vi "RT Main v1.0.vi"() -> ()   [LabVIEW 2017]
doc: "Changelog:\n\nv0.9:\n- Autocycle"
uses:
  Controls/Auto Delays.ctl
  support/Controls/All Inputs.ctl
  support/Controls/Index Details.ctl
  support/Controls/Auto Stats.ctl
  Controls/Auto Times.ctl
  Global Variables/RT GV.vi
  support/Message Queue/Enqueue Message (Single).vi
  Global Variables/FPGA GV.vi
  <vilib>/Utility/error.llb/Error Cluster From Error Code.vi
  <vilib>/rvi/errors/niLvFpgaAdjustHostInterfaceError.vi
  Global Variables/Network Globals.vi
  <vilib>/FPGAPlugInAG/Dynamic/niLvFpga_Close_Dynamic.vi
  <vilib>/rvi/interface/nirviReadWriteControl/nirviReadWriteControl.xnode
  Controls/FPGA Ref.ctl
  <vilib>/rvi/interface/nirviCloseFPGA/nirviCloseFPGA.xnode
  support/Message Queue/Message Queue.lvlib
  NiFpgaLv.dll
  <vilib>/rvi/interface/Simulation/niFpgaSimulationCallBeginRW.vi
panel:
  in  "Auto Para":T1={"Agitator Delays"=[250, 350], "TF Delays"=[700, 800, 2], "Insertion Delays"=[100, 500], "Cutting Delays"=[300, 300, 100], "PF Delays"=[250, 30000], "Measur. Delays"=[500.0, 188.9, 1.0], "Reject Delays"=[500], "BF Delays"=[1000, 1000]}
  in  "Stop Button 4":bool
  out "error out":errorcluster
  out "Wrong Message":string
  in  "Stop Button":bool
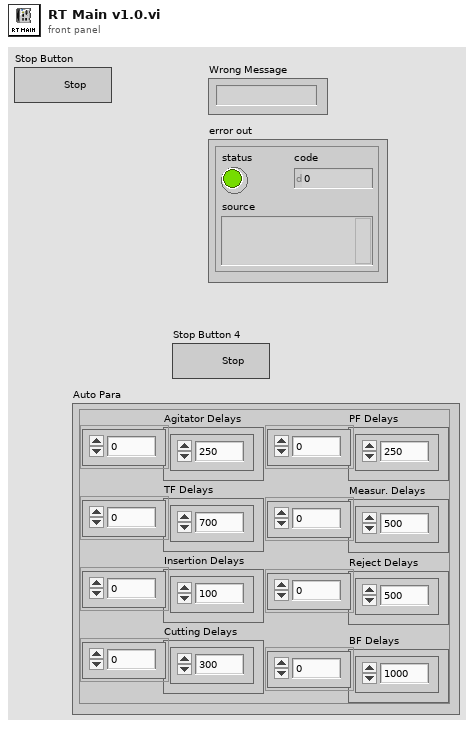
[diagram p1: front panel]
types:
  T1 = typedef "Auto Delays.ctl" = cluster{"Agitator Delays":u32[], "TF Delays":u32[], "Insertion Delays":u32[], "Cutting Delays":u32[], "PF Delays":u32[], "Measur. Delays":dbl[], "Reject Delays":u32[], "BF Delays":u32[]}
  T2 = typedef "FPGA Ref.ctl" = refnum<k20>
  T3 = cluster{"TL_Red":bool, "TL_Orange":bool, "TL_Green":bool, "TL_Buzzer":bool, "SOL_Index_Rotary_CW":bool, "SOL_Index_CNVR_Rotary_CCW":bool, "SOL_Index_CNVR_Stopper_Rear":bool, "SOL_Index_CNVR_Output _Separator _Rear":bool, "Bowl  Feeder_ ON":bool, "Pump_CNVR_Motor _ON":bool, "SOL_Gating_CYL_Rear":bool, "SOL_Tube_Feed_Agitatator":bool, "SOL_Tube_Feed_Gating_CYL":bool, "SOL_Insertion _CYL":bool, "SOL_Insertion_Clamp_CYL":bool, "SOL_Cutting_CYL":bool, "SOL_Cutting_Clamp_CYL":bool, "SOL_Insertion_Air_Nozzle":bool, "SOL_Measurement_CYL":bool, "SOL_Measure_Clamp_CYL":bool, "SOL_Rejection CYL_1":bool, "SOL_Rejection CYL_2":bool, "SOL_Rejection CYL_3":bool, "SOL_Rejection CYL_4":bool, "DO1.24":bool, "DO1.25":bool, "DO1.26":bool, "DO1.27":bool, "DO1.28":bool, "DO1.29":bool, "DO1.30":bool, "DO1.31":bool}
  T4 = typedef "All Inputs.ctl" = cluster{"DI 1":cluster{"Machine_ON":bool, "E_stop ":bool, "SW_Pressure":bool, "SW_Start ":bool, "SW_Reset":bool, "SW_Stop":bool, "SW_Door":bool, "RS_Index_Rotary_CW":bool, "RS_Index_Rotary_CCW":bool, "RS_Index_Stopper _Rear":bool, "RS_Index_Output_Separator_Rear":bool, "PES_Index_Pallet_Sensor":bool, "PES_Index_Output_Part Sensor":bool, "ICS_BF_Low_Level_1":bool, "ICS_BF_Low_Level_2":bool, "ICS_BF_Pump_CNVR_Full_1":bool, "ICS_BF_Pump_CNVR_Full_2":bool, "ICS_BF_Pump_CNVR_Full_3":bool, "ICS_BF_Pump_CNVR_Full_4":bool, "PES_PC_Pump Presence_1":bool, "PES_PC_Pump Presence_2":bool, "PES_PC_Pump Presence_3":bool, "PES_PC_Pump Presence_4":bool, "RS_PC_Gating_Front":bool, "PES_Pump_Interference":bool, "PES_TF_Low_Level":bool, "PES_Tube Presence_1":bool, "PES_Tube Presence_2":bool, "PES_Tube Presence_3":bool, "PES_Tube Presence_4":bool, "DI1.30":bool, "DI1.31":bool}, "DI 2":cluster{"RS_Agitatator_1_Rear ":bool, "RS_Agitatator_2_Rear ":bool, "RS_TF_Gating CYL_Rear":bool, "RS_Insertion_1_Rear":bool, "RS_Insertion_1_Front":bool, "RS_Insertion _2_Rear":bool, "RS_Insertion _2_Front":bool, "RS_Insertion _3_Rear":bool, "RS_Insertion _3_Front":bool, "RS_Insertion _4_Rear":bool, "RS_Insertion _4_Front":bool, "RS_Insertion_Clamp_Rear":bool, "RS_Cutting_Rear":bool, "RS_Cutting_Clamp _Rear":bool, "RS_Measurement_1_Rear":bool, "RS_Measurement_2_Rear":bool, "RS_Measurement_3_Rear":bool, "RS_Measurement_4_Rear":bool, "RS_Measure_Clamp_Rear":bool, "RS_Rejection_1_Rear":bool, "RS_Rejection_2_Rear":bool, "RS_Rejection_3_Rear":bool, "RS_Rejection_4_Rear":bool, "DI2.23":bool, "DI2.24":bool, "DI2.25":bool, "DI2.26":bool, "DI2.27":bool, "DI2.28":bool, "DI2.29":bool, "DI2.30":bool, "DI2.31":bool}, "IAS 1":dbl, "IAS 2":dbl, "IAS 3":dbl, "IAS 4":dbl, "DO 1":cluster{"TL_Red":bool, "TL_Orange":bool, "TL_Green":bool, "TL_Buzzer":bool, "SOL_Index_Rotary_CW":bool, "SOL_Index_CNVR_Rotary_CCW":bool, "SOL_Index_CNVR_Stopper_Rear":bool, "SOL_Index_CNVR_Output _Separator _Rear":bool, "Bowl  Feeder_ ON 1":bool, "Pump_CNVR_Motor _ON":bool, "SOL_PC_Gating_CYL_Rear":bool, "SOL_Tube_Feed_Agitatator":bool, "SOL_Tube_Feed_Gating_CYL":bool, "SOL_Insertion _CYL":bool, "SOL_Insertion_Clamp_CYL":bool, "SOL_Cutting_CYL":bool, "SOL_Cutting_Clamp_CYL":bool, "SOL_Insertion_Air_Nozzle":bool, "SOL_Measurement_CYL":bool, "DO1.19":bool, "SOL_Rejection CYL_1":bool, "SOL_Rejection CYL_2":bool, "SOL_Rejection CYL_3":bool, "SOL_Rejection CYL_4":bool, "Bowl  Feeder_ ON 2":bool, "SOL_BF_BlowerON":bool, "SOL_BF1_Track1":bool, "SOL_BF1_Track2":bool, "SOL_BF2_Track1":bool, "SOL_BF2_Track2":bool, "DO1.30":bool, "DO1.31":bool}}
  T5 = typedef "Index Details.ctl" = cluster{"Time (ms)":u32, "Waveform Graph":i16[]}
  T6 = cluster{T1, "Reject Pallets":cluster{"Reject 1":bool, "Reject 2":bool, "Reject 3":bool, "Reject 4":bool}}
  T7 = typedef "Auto Stats.ctl" = cluster{"Time-Stamp":timestamp, "Auto Times":T8, "Measurements":cluster{"1":dbl, "2":dbl, "3":dbl, "4":dbl}, "Outputs":cluster{"Good Parts":u32, "Reject Parts":u32}, "Cycle Time":dbl, "Remarks":string}
  T8 = typedef "Auto Times.ctl" = cluster{"Index Time":u32, "TF Time":u32, "Insertion Time":u32, "Cutting Time":u32, "PF Time":u32, "Meas. Time":u32, "Reject Time":u32}
  T9 = cluster{"TL_Red":bool, "TL_Orange":bool, "TL_Green":bool, "TL_Buzzer":bool, "SOL_Index_Rotary_CW":bool, "SOL_Index_CNVR_Rotary_CCW":bool, "SOL_Index_CNVR_Stopper_Rear":bool, "SOL_Index_CNVR_Output _Separator _Rear":bool, "Bowl Feeder_ ON1":bool, "Pump_CNVR_Motor _ON":bool, "SOL_PC_Gating_CYL_Rear":bool, "SOL_Tube_Feed_Agitatator":bool, "SOL_Tube_Feed_Gating_CYL":bool, "SOL_Insertion _CYL":bool, "SOL_Insertion_Clamp_CYL":bool, "SOL_Cutting_CYL":bool, "SOL_Cutting_Clamp_CYL":bool, "SOL_Insertion_Air_Nozzle":bool, "SOL_Measurement_CYL":bool, "DO1.19":bool, "SOL_Rejection CYL_1":bool, "SOL_Rejection CYL_2":bool, "SOL_Rejection CYL_3":bool, "SOL_Rejection CYL_4":bool, "Bowl Feeder_ON2":bool, "SOL_BF_BlowerON":bool, "SOL_BF1_Track1":bool, "SOL_BF1_Track2":bool, "SOL_BF2_Track1":bool, "SOL_BF2_Track2":bool, "DO1.30":bool, "DO1.31":bool}
  T10 = cluster{"Machine_ON":bool, "E_stop ":bool, "SW_Pressure":bool, "SW_Start ":bool, "SW_Reset":bool, "SW_Stop":bool, "SW_Door":bool, "RS_Index_Rotary_CW":bool, "RS_Index_Rotary_CCW":bool, "RS_Index_Stopper _Rear":bool, "RS_Index_Output_Separator_Rear":bool, "PES_Index_Pallet_Sensor":bool, "PES_Index_Output_Part Sensor":bool, "ICS_BF_Low_Level_1":bool, "ICS_BF_Low_Level_2":bool, "ICS_BF_Pump_CNVR_Full_1":bool, "ICS_BF_Pump_CNVR_Full_2":bool, "ICS_BF_Pump_CNVR_Full_3":bool, "ICS_BF_Pump_CNVR_Full_4":bool, "PES_PC_Pump Presence_1":bool, "PES_PC_Pump Presence_2":bool, "PES_PC_Pump Presence_3":bool, "PES_PC_Pump Presence_4":bool, "RS_PC_Gating_Front":bool, "PES_Pump_Interference":bool, "PES_TF_Low_Level":bool, "PES_Tube Presence_1":bool, "PES_Tube Presence_2":bool, "PES_Tube Presence_3":bool, "PES_Tube Presence_4":bool, "DI1.30":bool, "DI1.31":bool}
  T11 = cluster{"RS_Agitatator_1_Rear ":bool, "RS_Agitatator_2_Rear ":bool, "RS_TF_Gating CYL_Rear":bool, "RS_Insertion_1_Rear":bool, "RS_Insertion_1_Front":bool, "RS_Insertion _2_Rear":bool, "RS_Insertion _2_Front":bool, "RS_Insertion _3_Rear":bool, "RS_Insertion _3_Front":bool, "RS_Insertion _4_Rear":bool, "RS_Insertion _4_Front":bool, "RS_Insertion_Clamp_Rear":bool, "RS_Cutting_Rear":bool, "RS_Cutting_Clamp _Rear":bool, "RS_Measurement_1_Rear":bool, "RS_Measurement_2_Rear":bool, "RS_Measurement_3_Rear":bool, "RS_Measurement_4_Rear":bool, "DI2.18":bool, "RS_Rejection_1_Rear":bool, "RS_Rejection_2_Rear":bool, "RS_Rejection_3_Rear":bool, "RS_Rejection_4_Rear":bool, "DI2.23":bool, "DI2.24":bool, "DI2.25":bool, "DI2.26":bool, "DI2.27":bool, "DI2.28":bool, "DI2.29":bool, "DI2.30":bool, "DI2.31":bool}
  T12 = cluster{"Array":string[][], "Machine Status":string}
  T13 = cluster{"Measurements":cluster{"1":dbl, "2":dbl, "3":dbl, "4":dbl}, "Reject Pallets":cluster{"Reject 1":bool, "Reject 2":bool, "Reject 3":bool, "Reject 4":bool}}
  T14 = cluster{"Auto Times":T8, "Results":cluster{"Measurements":cluster{"1":dbl, "2":dbl, "3":dbl, "4":dbl}, "Reject Pallets":cluster{"Reject 1":bool, "Reject 2":bool, "Reject 3":bool, "Reject 4":bool}}, "OutputCount":u32, "error out":errorcluster}
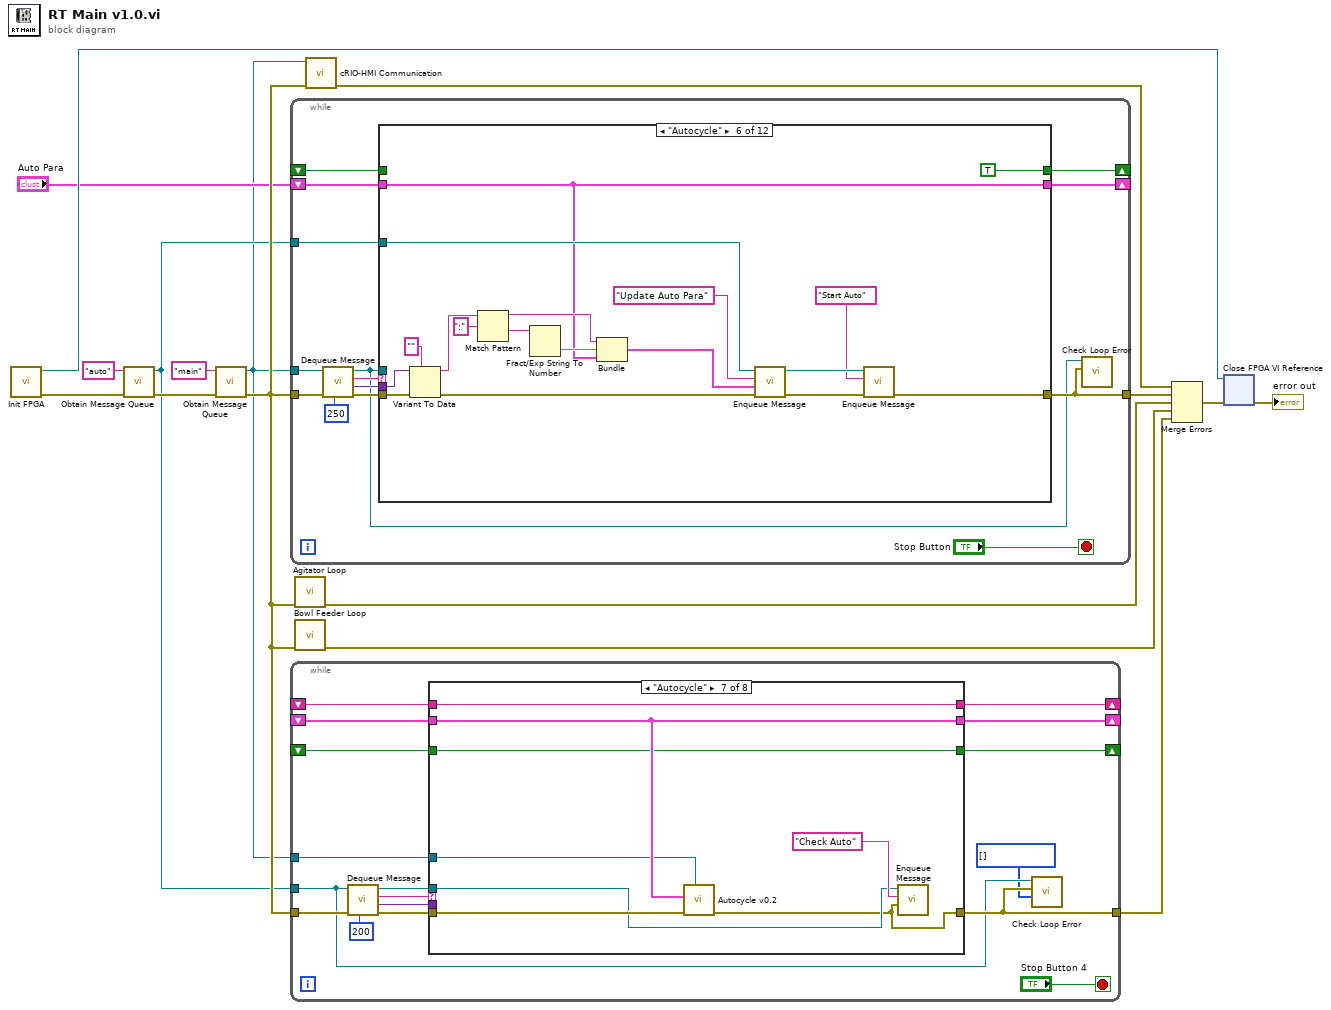
[diagram p0: block diagram]
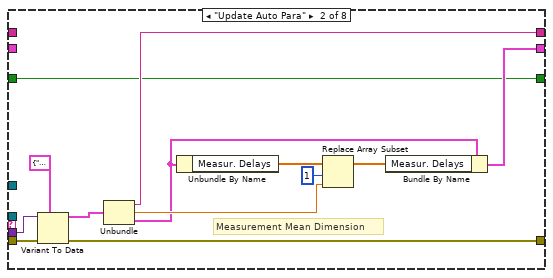
[diagram p3: hidden frame]
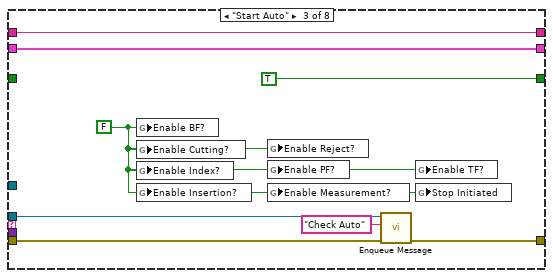
[diagram p4: hidden frame]
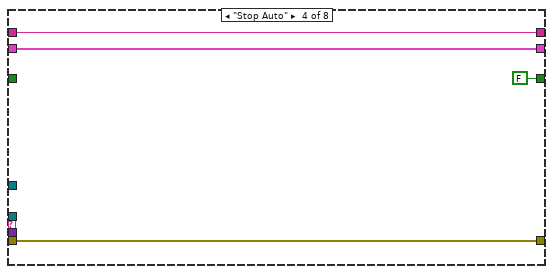
[diagram p5: hidden frame]
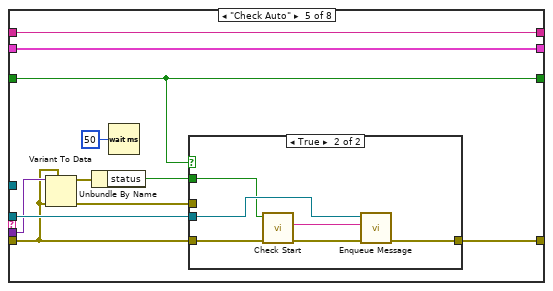
[diagram p6: hidden frame]
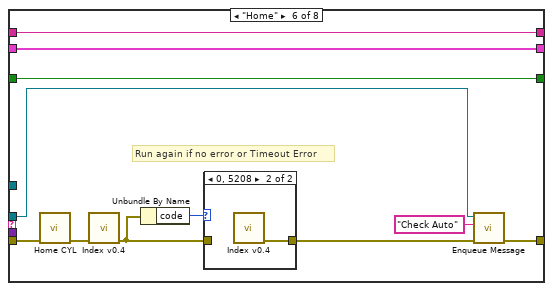
[diagram p8: hidden frame]
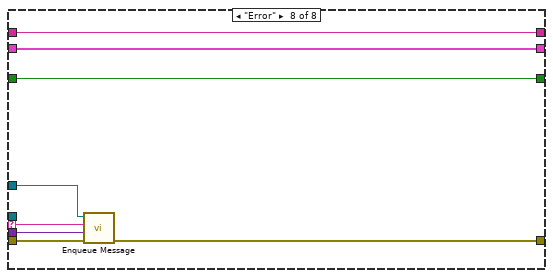
[diagram p10: hidden frame]
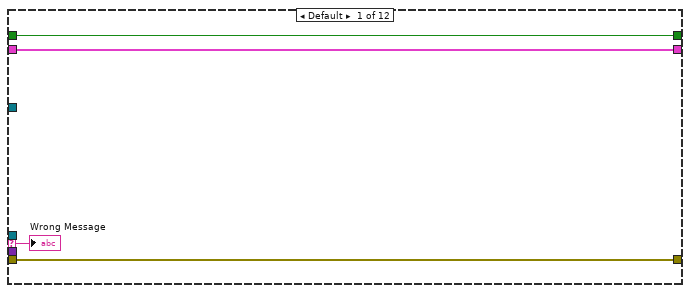
[diagram p11: hidden frame]
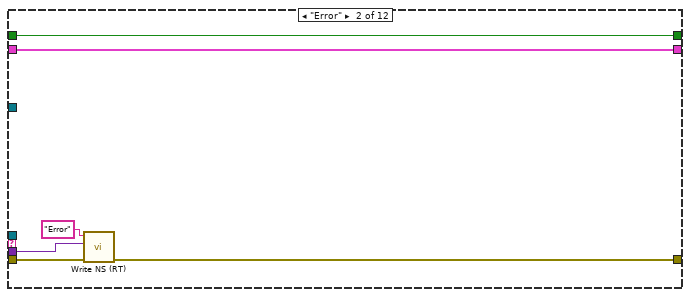
[diagram p12: hidden frame]
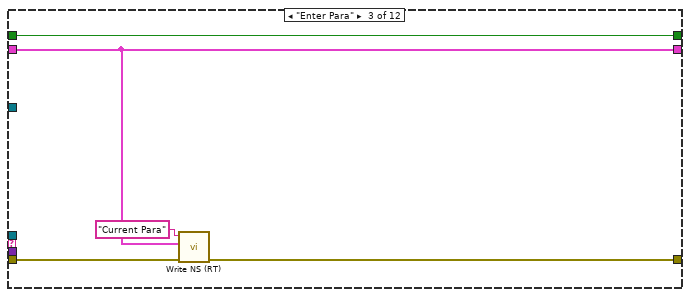
[diagram p13: hidden frame]
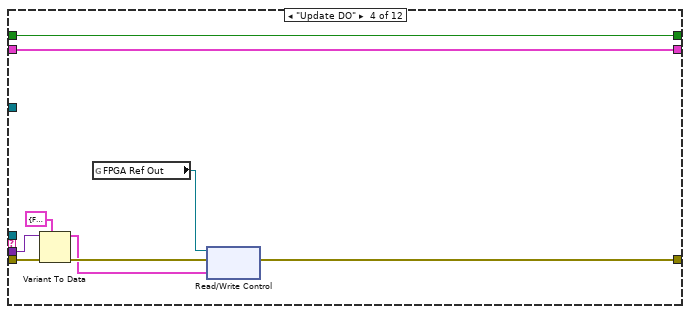
[diagram p14: hidden frame]
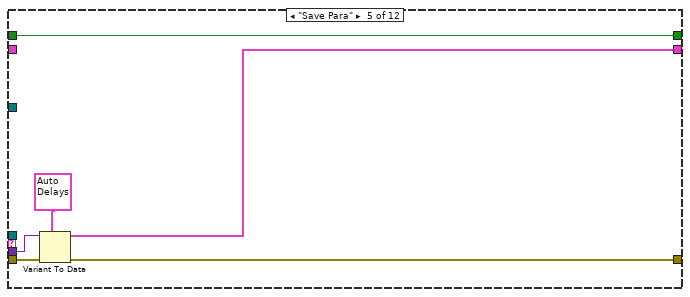
[diagram p15: hidden frame]
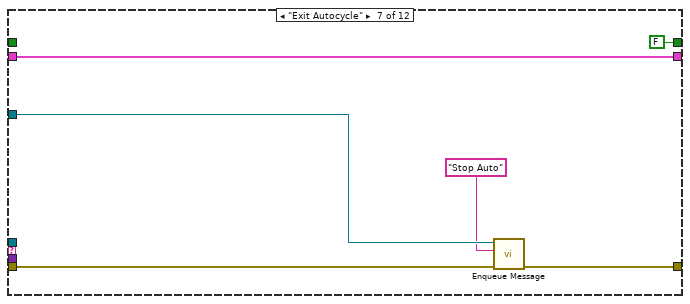
[diagram p16: hidden frame]
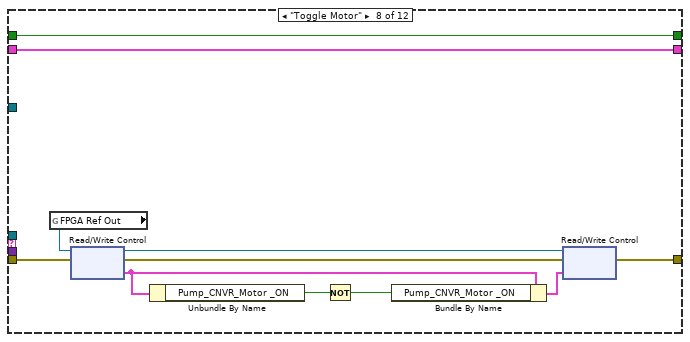
[diagram p17: hidden frame]
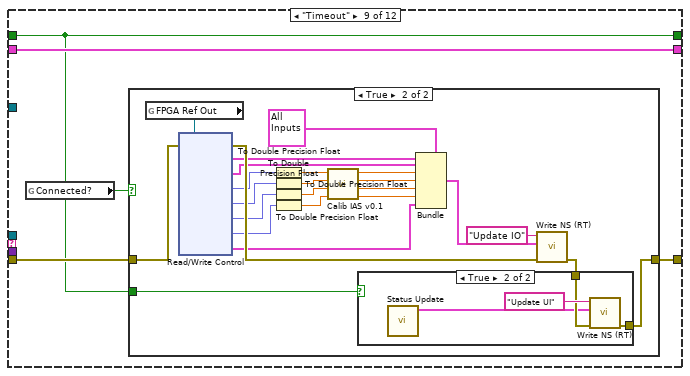
[diagram p18: hidden frame]
diagram:
  n1 = call "Init FPGA.vi"() -> ("error out"=w5:errorcluster, "FPGA Ref Out"=w10:T2)  [unwired: 10 in]
  n2 = call "Obtain Message Queue.vi"("error in (no error)"=w5, "name"="auto") -> ("error out"=w4:errorcluster, "Message Queue"=w2:refnum<queue>)  [unwired: 8 in]
  n3 = call "Obtain Message Queue.vi"("error in (no error)"=w4, "name"="main") -> ("error out"=w9:errorcluster, "Message Queue"=w1:refnum<queue>)  [unwired: 8 in]
  n4 = while {
    tunnel: w9 -> [w29]
    tunnel: w1 -> [w28]
    tunnel: [w24] -> w16
    tunnel: w2 -> [w21]
    shift-right: [w19] -> _
    shift-left: "Auto Para" -> [w20]
    shift-right: [w17] -> _
    shift-left: _ -> [w18]
    stop <- "Stop Button" stop-if-true
    n5 = call "Dequeue Message.vi"("timeout"=250, "error in (no error)"=w29, "Message Queue"=w28) -> ("error out"=w27:errorcluster, "Message Data"=w25:variant, "Message"=w26:string, "dup Message Queue"=w23:refnum<queue>)  [unwired: 5 in]
    n6 = case shown="\"Autocycle\"" w26 {
      selector: w26 -> [w34 _ _ _ _ _ _ _ _ _ _ _]
      tunnel: w27 -> [w33 w39 w45 w54 w60 w78 w84 w94 w99 w142 w169 w179]
      tunnel: w23 -> [_ _ _ _ _ _ _ _ _ w134 _ _]
      tunnel: w25 -> [_ w37 _ w53 w59 w77 _ _ _ _ w168 w178]
      tunnel: [w33 w38 w44 w49 w58 w64 w81 w92 w100 w135 w164 w175] -> w24
      tunnel: w21 -> [_ _ _ _ _ w70 w83 _ _ _ _ _]
      tunnel: w20 -> [w32 w40 w42 w47 _ w67 w82 w86 w97 w132 w155 w174]
      tunnel: [w32 w40 w42 w47 w57 w67 w82 w86 w97 w132 w155 w174] -> w19
      tunnel: w18 -> [w31 w35 w41 w46 w55 _ _ w85 w96 w131 w152 w170]
      tunnel: [w31 w35 w41 w46 w55 TRUE FALSE w85 w96 w131 w152 w170] -> w17
      frame Default {
        "Wrong Message" <- w34
      }
      frame "Error" {
        n7 = call "Write NS (RT).vi"("error in (no error)"=w39, "Message Data"=w37, "Message"="Error") -> ("error out"=w38:errorcluster)  [unwired: 8 in]
      }
      frame "Enter Para" {
        n8 = call "Write NS (RT).vi"("error in (no error)"=w45, "Message Data"=w42, "Message"="Current Para") -> ("error out"=w44:errorcluster)  [unwired: 8 in]
      }
      frame "Update DO" {
        n9 = Variant To Data(error in=w54, type=T3 {"TL_Red"=FALSE, "TL_Orange"=FALSE, "TL_Green"=FALSE, "TL_Buzzer"=FALSE, "SOL_Index_Rotary_CW"=FALSE, "SOL_Index_CNVR_Rotary_CCW"=FALSE, "SOL_Index_CNVR_Stopper_Rear"=FALSE, "SOL_Index_CNVR_Output _Separator _Rear"=FALSE, "Bowl  Feeder_ ON"=FALSE, "Pump_CNVR_Motor _ON"=FALSE, "SOL_Gating_CYL_Rear"=FALSE, "SOL_Tube_Feed_Agitatator"=FALSE, "SOL_Tube_Feed_Gating_CYL"=FALSE, "SOL_Insertion _CYL"=FALSE, "SOL_Insertion_Clamp_CYL"=FALSE, "SOL_Cutting_CYL"=FALSE, "SOL_Cutting_Clamp_CYL"=FALSE, "SOL_Insertion_Air_Nozzle"=FALSE, "SOL_Measurement_CYL"=FALSE, "SOL_Measure_Clamp_CYL"=FALSE, "SOL_Rejection CYL_1"=FALSE, "SOL_Rejection CYL_2"=FALSE, "SOL_Rejection CYL_3"=FALSE, "SOL_Rejection CYL_4"=FALSE, "DO1.24"=FALSE, "DO1.25"=FALSE, "DO1.26"=FALSE, "DO1.27"=FALSE, "DO1.28"=FALSE, "DO1.29"=FALSE, "DO1.30"=FALSE, "DO1.31"=FALSE} ("DO 1"), Variant=w53) -> (data=w48:T3, error out=w50:errorcluster)
        n10 = global read "FPGA GV.vi" "FPGA Ref Out"() -> (w51:T2)
        n11 = xnode "Read/Write Control"("FPGA VI Reference In"=w51, "error in"=w50, "DO 1"=w48) -> ("error out"=w49:errorcluster)  [unwired: 1 out]
      }
      frame "Save Para" {
        n12 = Variant To Data(error in=w60, type=T1 {"Agitator Delays"=[700, 250], "TF Delays"=[700, 800, 2], "Insertion Delays"=[100, 500], "Cutting Delays"=[300, 300, 100], "PF Delays"=[250, 30000], "Measur. Delays"=[500.0, 188.9, 1.0], "Reject Delays"=[500], "BF Delays"=[1000, 1000]} ("Auto Para"), Variant=w59) -> (data=w57:T1, error out=w58:errorcluster)
      }
      frame "Autocycle" {
        n13 = Variant To Data(error in=w78, type="", Variant=w77) -> (data=w73:string, error out=w71:errorcluster)
        n14 = Match Pattern(string=w73, regular expression=":") -> (before substring=w69:string, after substring=w74:string)  [unwired: 1 in, 2 out]
        n15 = Fract/Exp String To Number(string=w74) -> (number=w68:dbl)  [unwired: 3 in, 1 out]
        n16 = Bundle(w69, w68, "Auto Para"=w67) -> (w66:cluster{string, dbl, "Auto Para":T1})  [unwired: 1 in]
        n17 = call-poly "Enqueue Message.vi"("error in (no error)"=w71, "Message Data"=w66, "Message"="Update Auto Para", "Message Queue"=w70) -> ("error out"=w65:errorcluster, "dup Message Queue"=w63:refnum<queue>)  [unwired: 6 in]
        n18 = call-poly "Enqueue Message.vi"("error in (no error)"=w65, "Message"="Start Auto", "Message Queue"=w63) -> ("error out"=w64:errorcluster)  [unwired: 7 in, 1 out]
      }
      frame "Exit Autocycle" {
        n19 = call-poly "Enqueue Message.vi"("error in (no error)"=w84, "Message"="Stop Auto", "Message Queue"=w83) -> ("error out"=w81:errorcluster)  [unwired: 7 in, 1 out]
      }
      frame "Toggle Motor" {
        n20 = global read "FPGA GV.vi" "FPGA Ref Out"() -> (w95:T2)
        n21 = xnode "Read/Write Control"("FPGA VI Reference In"=w95, "error in"=w94) -> ("FPGA VI Reference Out"=w91:T2, "error out"=w93:errorcluster, "DO 1"=w89:T9)
        n22 = Unbundle By Name(w89) -> ("Pump_CNVR_Motor _ON"=w90:bool)
        n23 = Not(x=w90) -> (.not. x?=w87:bool)
        n24 = Bundle By Name(cluster=w89, "Pump_CNVR_Motor _ON"=w87) -> (w88:T9)
        n25 = xnode "Read/Write Control"("FPGA VI Reference In"=w91, "error in"=w93, "DO 1"=w88) -> ("error out"=w92:errorcluster)  [unwired: 1 out]
      }
      frame "Timeout" {
        n26 = global read "Network Globals.vi" "Connected?"() -> (w98:bool)
        n27 = case shown="True" w98 {
          tunnel: [w101 w104] -> w100
          tunnel: w99 -> [w101 w124]
          tunnel: w96 -> [_ w102]
          frame False {
          }
          frame True {
            n28 = global read "FPGA GV.vi" "FPGA Ref Out"() -> (w103:T2)
            n29 = xnode "Read/Write Control"("FPGA VI Reference In"=w103, "error in"=w124) -> ("error out"=w123:errorcluster, "DI 1"=w122:T10, "DI 2"=w121:T11, "AI0"=w120:fxp<+/-,27,6>, "AI1"=w119:fxp<+/-,27,6>, "AI2"=w118:fxp<+/-,27,6>, "AI3"=w117:fxp<+/-,27,6>, "DO 1"=w114:T9)  [unwired: 1 out]
            n30 = To Double Precision Float(number=w120) -> (double precision float=w107:dbl)
            n31 = To Double Precision Float(number=w119) -> (double precision float=w109:dbl)
            n32 = To Double Precision Float(number=w118) -> (double precision float=w111:dbl)
            n33 = To Double Precision Float(number=w117) -> (double precision float=w113:dbl)
            n34 = call "Calib IAS v0.1.vi"("x 4"=w113, "x 3"=w111, "x 2"=w109, "x"=w107) -> ("y 4"=w112:dbl, "y 3"=w110:dbl, "y 2"=w108:dbl, "y 1"=w106:dbl)  [unwired: 2 in, 2 out]
            n35 = Bundle(cluster=T4 {"DI 1"={"Machine_ON"=FALSE, "E_stop "=FALSE, "SW_Pressure"=FALSE, "SW_Start "=FALSE, "SW_Reset"=FALSE, "SW_Stop"=FALSE, "SW_Door"=FALSE, "RS_Index_Rotary_CW"=FALSE, "RS_Index_Rotary_CCW"=FALSE, "RS_Index_Stopper _Rear"=FALSE, "RS_Index_Output_Separator_Rear"=FALSE, "PES_Index_Pallet_Sensor"=FALSE, "PES_Index_Output_Part Sensor"=FALSE, "ICS_BF_Low_Level_1"=FALSE, "ICS_BF_Low_Level_2"=FALSE, "ICS_BF_Pump_CNVR_Full_1"=FALSE, "ICS_BF_Pump_CNVR_Full_2"=FALSE, "ICS_BF_Pump_CNVR_Full_3"=FALSE, "ICS_BF_Pump_CNVR_Full_4"=FALSE, "PES_PC_Pump Presence_1"=FALSE, "PES_PC_Pump Presence_2"=FALSE, "PES_PC_Pump Presence_3"=FALSE, "PES_PC_Pump Presence_4"=FALSE, "RS_PC_Gating_Front"=FALSE, "PES_Pump_Interference"=FALSE, "PES_TF_Low_Level"=FALSE, "PES_Tube Presence_1"=FALSE, "PES_Tube Presence_2"=FALSE, "PES_Tube Presence_3"=FALSE, "PES_Tube Presence_4"=FALSE, "DI1.30"=FALSE, "DI1.31"=FALSE}, "DI 2"={"RS_Agitatator_1_Rear "=FALSE, "RS_Agitatator_2_Rear "=FALSE, "RS_TF_Gating CYL_Rear"=FALSE, "RS_Insertion_1_Rear"=FALSE, "RS_Insertion_1_Front"=FALSE, "RS_Insertion _2_Rear"=FALSE, "RS_Insertion _2_Front"=FALSE, "RS_Insertion _3_Rear"=FALSE, "RS_Insertion _3_Front"=FALSE, "RS_Insertion _4_Rear"=FALSE, "RS_Insertion _4_Front"=FALSE, "RS_Insertion_Clamp_Rear"=FALSE, "RS_Cutting_Rear"=FALSE, "RS_Cutting_Clamp _Rear"=FALSE, "RS_Measurement_1_Rear"=FALSE, "RS_Measurement_2_Rear"=FALSE, "RS_Measurement_3_Rear"=FALSE, "RS_Measurement_4_Rear"=FALSE, "RS_Measure_Clamp_Rear"=FALSE, "RS_Rejection_1_Rear"=FALSE, "RS_Rejection_2_Rear"=FALSE, "RS_Rejection_3_Rear"=FALSE, "RS_Rejection_4_Rear"=FALSE, "DI2.23"=FALSE, "DI2.24"=FALSE, "DI2.25"=FALSE, "DI2.26"=FALSE, "DI2.27"=FALSE, "DI2.28"=FALSE, "DI2.29"=FALSE, "DI2.30"=FALSE, "DI2.31"=FALSE}, "IAS 1"=0.0, "IAS 2"=0.0, "IAS 3"=0.0, "IAS 4"=0.0, "DO 1"={"TL_Red"=FALSE, "TL_Orange"=FALSE, "TL_Green"=FALSE, "TL_Buzzer"=FALSE, "SOL_Index_Rotary_CW"=FALSE, "SOL_Index_CNVR_Rotary_CCW"=FALSE, "SOL_Index_CNVR_Stopper_Rear"=FALSE, "SOL_Index_CNVR_Output _Separator _Rear"=FALSE, "Bowl  Feeder_ ON 1"=FALSE, "Pump_CNVR_Motor _ON"=FALSE, "SOL_PC_Gating_CYL_Rear"=FALSE, "SOL_Tube_Feed_Agitatator"=FALSE, "SOL_Tube_Feed_Gating_CYL"=FALSE, "SOL_Insertion _CYL"=FALSE, "SOL_Insertion_Clamp_CYL"=FALSE, "SOL_Cutting_CYL"=FALSE, "SOL_Cutting_Clamp_CYL"=FALSE, "SOL_Insertion_Air_Nozzle"=FALSE, "SOL_Measurement_CYL"=FALSE, "DO1.19"=FALSE, "SOL_Rejection CYL_1"=FALSE, "SOL_Rejection CYL_2"=FALSE, "SOL_Rejection CYL_3"=FALSE, "SOL_Rejection CYL_4"=FALSE, "Bowl  Feeder_ ON 2"=FALSE, "SOL_BF_BlowerON"=FALSE, "SOL_BF1_Track1"=FALSE, "SOL_BF1_Track2"=FALSE, "SOL_BF2_Track1"=FALSE, "SOL_BF2_Track2"=FALSE, "DO1.30"=FALSE, "DO1.31"=FALSE}}, "DI 1"=w122, "DI 2"=w121, "IAS 1"=w106, "IAS 2"=w108, "IAS 3"=w110, "IAS 4"=w112, "DO 1"=w114) -> (w116:T4)
            n36 = call "Write NS (RT).vi"("error in (no error)"=w123, "Message Data"=w116, "Message"="Update IO") -> ("error out"=w105:errorcluster)  [unwired: 8 in]
            n37 = case shown="True" w102 {
              tunnel: w105 -> [w126 w129]
              tunnel: [w126 w128] -> w104
              frame False {
              }
              frame True {
                n38 = call "Status Update.vi"() -> ("Status Cluster"=w127:T12)  [unwired: 11 in]
                n39 = call "Write NS (RT).vi"("error in (no error)"=w129, "Message Data"=w127, "Message"="Update UI") -> ("error out"=w128:errorcluster)  [unwired: 8 in]
              }
            }
          }
        }
      }
      frame "Manual Index" {
        n40 = call "Index v0.4.vi"("error in (no error)"=w142) -> ("error out"=w140:errorcluster, "Waveform Graph"=w138:i16[], "Index Time"=w139:u32)  [unwired: 7 in, 1 out]
        n41 = Bundle(cluster=T5 {"Time (ms)"=0, "Waveform Graph"=[]}, "Time (ms)"=w139, "Waveform Graph"=w138) -> (w137:T5)
        n42 = call "Write NS (RT).vi"("error in (no error)"=w140, "Message Data"=w137, "Message"="Update Index") -> ("error out"=w136:errorcluster)  [unwired: 8 in]
        n43 = flat-sequence {
          tunnel: w136 -> [w146]
          tunnel: [w145] -> w135
          tunnel: w134 -> [w143]
          frame #0 {
            n44 = global read "RT GV.vi" "Continuous Index?"() -> (w144:bool)
            n45 = case shown="True" w144 {
              tunnel: w146 -> [w147 w151]
              tunnel: [w147 w150] -> w145
              tunnel: w143 -> [_ w148]
              frame False {
              }
              frame True {
                n46 = call-poly "Enqueue Message.vi"("error in (no error)"=w151, "Message"="Manual Index", "Message Queue"=w148) -> ("error out"=w150:errorcluster)  [unwired: 7 in, 1 out]
              }
            }
          }
        }
      }
      frame "Manual Run" {
        n47 = Variant To Data(error in=w169, type=T6 {{"Agitator Delays"=[1000], "TF Delays"=[1000], "Insertion Delays"=[1000], "Cutting Delays"=[1000], "PF Delays"=[1000], "Measur. Delays"=[1000.0], "Reject Delays"=[1000], "BF Delays"=[1000]}, "Reject Pallets"={"Reject 1"=FALSE, "Reject 2"=FALSE, "Reject 3"=FALSE, "Reject 4"=FALSE}}, Variant=w168) -> (data=w160:T6, error out=w167:errorcluster)
        n48 = Unbundle(w160) -> (w157:T1)  [unwired: 1 out]
        n49 = Unbundle By Name(w157) -> ("Agitator Delays"=w154:u32[], "BF Delays"=w153:u32[])
        n50 = call "Manual.vi"("error in"=w167, "Auto Delays"=w157) -> ("error out"=w159:errorcluster, "OutputCount"=w158:u32, "Results"=w156:T13, "Auto Times"=w163:T8)  [unwired: 6 in]
        n51 = global write "RT GV.vi" "Agitator Delays"(w154) -> ()
        n52 = global write "RT GV.vi" "BF Delays"(w153) -> ()
        n53 = Bundle("Auto Times"=w163, "Results"=w156, "OutputCount"=w158, "error out"=w159) -> (w162:T14)  [unwired: 1 in]
        n54 = call "Write NS (RT).vi"("Message Data"=w162, "Message"="Manual Status") -> ("error out"=w165:errorcluster)  [unwired: 9 in]
        n55 = Merge Errors(w165) -> (w164:errorcluster)
      }
      frame "Log Cycle" {
        n56 = Variant To Data(error in=w179, type=T7 {"Time-Stamp"=timestamp(0 s since 1904-01-01), "Auto Times"={"Index Time"=0, "TF Time"=0, "Insertion Time"=0, "Cutting Time"=0, "PF Time"=0, "Meas. Time"=0, "Reject Time"=0}, "Measurements"={"1"=0.0, "2"=0.0, "3"=0.0, "4"=0.0}, "Outputs"={"Good Parts"=0, "Reject Parts"=0}, "Cycle Time"=0.0, "Remarks"=""} ("Auto Stats"), Variant=w178) -> (data=w171:T7, error out=w172:errorcluster)
        n57 = call "Write NS (RT).vi"("error in (no error)"=w172, "Message Data"=w171, "Message"="Autocycle Log") -> ("error out"=w176:errorcluster)  [unwired: 8 in]
        n58 = Merge Errors(w176) -> (w175:errorcluster)
      }
    }
    n59 = call "Check Loop Error.vi"("error to process"=w24, "Message Queue"=w23) -> ()  [unwired: 8 in, 2 out]
  }
  n60 = while {
    tunnel: w9 -> [w194]
    tunnel: [w192] -> w8
    tunnel: w2 -> [w184]
    shift-right: [w188] -> _
    shift-left: _ -> [w187]
    shift-right: [w186] -> _
    shift-left: _ -> [w185]
    shift-right: [w183] -> _
    shift-left: _ -> [w182]
    tunnel: w1 -> [w181]
    stop <- "Stop Button 4" stop-if-true
    n61 = call "Dequeue Message.vi"("timeout"=200, "error in (no error)"=w194, "Message Queue"=w184) -> ("error out"=w193:errorcluster, "Message Data"=w189:variant, "Message"=w190:string, "dup Message Queue"=w191:refnum<queue>)  [unwired: 5 in]
    n62 = case shown="\"Autocycle\"" w190 {
      selector: w190 -> [_ _ _ _ _ _ _ w269]
      tunnel: w193 -> [w200 w213 w218 w223 w228 w251 w264 w267]
      tunnel: [w200 w212 w217 w223 w234 w246 w257 w266] -> w192
      tunnel: w191 -> [_ _ w216 _ w233 w244 w258 _]
      tunnel: w189 -> [_ w211 _ _ w230 _ _ w268]
      tunnel: [w199 w209 w221 w225 w236 w254 w263 w272] -> w188
      tunnel: w187 -> [w199 _ w221 w225 w236 w254 w263 w272]
      tunnel: [w198 w204 w220 w224 w235 w253 w262 w271] -> w186
      tunnel: w185 -> [w198 _ w220 w224 w235 w253 w262 w271]
      tunnel: [w197 w203 TRUE FALSE w232 w252 w260 w270] -> w183
      tunnel: w182 -> [w197 w203 _ _ w232 w252 w260 w270]
      tunnel: w181 -> [_ _ _ _ _ _ w261 w265]
      frame Default {
      }
      frame "Update Auto Para" {
        # "Measurement Mean Dimension"
        n63 = Variant To Data(error in=w213, type=cluster{string, dbl, "Auto Para":T1} {"", 0.0, "Auto Para"={"Agitator Delays"=[], "TF Delays"=[], "Insertion Delays"=[], "Cutting Delays"=[], "PF Delays"=[], "Measur. Delays"=[], "Reject Delays"=[], "BF Delays"=[]}} ("cluster"), Variant=w211) -> (data=w210:cluster{string, dbl, "Auto Para":T1}, error out=w212:errorcluster)
        n64 = Unbundle(w210) -> (w209:string, w206:dbl, "Auto Para"=w201:T1)
        n65 = Unbundle By Name(w201) -> ("Measur. Delays"=w208:dbl[])
        n66 = Replace Array Subset(array=w208, new element=w206, index=1) -> (w205:dbl[])
        n67 = Bundle By Name(cluster=w201, "Measur. Delays"=w205) -> (w204:T1)
      }
      frame "Start Auto" {
        w214 = FALSE ("Enable BF?")
        n68 = global write "RT GV.vi" "Enable BF?"(w214) -> ()
        n69 = global write "RT GV.vi" "Enable Cutting?"(w214) -> ()
        n70 = global write "RT GV.vi" "Enable Index?"(w214) -> ()
        n71 = global write "RT GV.vi" "Enable Insertion?"(w214) -> ()
        n72 = global write "RT GV.vi" "Enable Reject?"(w214) -> ()
        n73 = global write "RT GV.vi" "Enable PF?"(w214) -> ()
        n74 = global write "RT GV.vi" "Enable Measurement?"(w214) -> ()
        n75 = call-poly "Enqueue Message.vi"("error in (no error)"=w218, "Message"="Check Auto", "Message Queue"=w216) -> ("error out"=w217:errorcluster)  [unwired: 7 in, 1 out]
        n76 = global write "RT GV.vi" "Enable TF?"(w214) -> ()
        n77 = global write "RT GV.vi" "Stop Initiated"(w214) -> ()
      }
      frame "Stop Auto" {
      }
      frame "Check Auto" {
        n78 = Variant To Data(error in=w228, type=w228, Variant=w230) -> (data=w227:errorcluster, error out=w229:errorcluster)
        n79 = Unbundle By Name(w227) -> ("status"=w226:bool)
        n80 = Wait (ms)(milliseconds to wait=u32 50) -> ()  [unwired: 1 out]
        n81 = case shown="True" w232 {
          tunnel: [w237 w243] -> w234
          tunnel: w233 -> [_ w239]
          tunnel: w228 -> [w237 w242]
          tunnel: w229 -> [_ _]
          tunnel: w226 -> [_ w238]
          frame False {
          }
          frame True {
            n82 = call "Check Start.vi"("error in"=w242, "Error Stop?"=w238) -> ("error out"=w241:errorcluster, "Message"=w240:string)  [unwired: 8 in]
            n83 = call-poly "Enqueue Message.vi"("error in (no error)"=w241, "Message"=w240, "Message Queue"=w239) -> ("error out"=w243:errorcluster)  [unwired: 7 in, 1 out]
          }
        }
      }
      frame "Home" {
        # "Run again if no error or Timeout Error"
        n84 = call "Home CYL.vi"("error in"=w251) -> ("error out"=w250:errorcluster)  [unwired: 10 in]
        n85 = call "Index v0.4.vi"("error in (no error)"=w250) -> ("error out"=w248:errorcluster)  [unwired: 7 in, 3 out]
        n86 = Unbundle By Name(w248) -> ("code"=w249:i32)
        n87 = case shown="0, 5208" w249 {
          tunnel: [w255 w256] -> w245
          tunnel: w248 -> [w255 _]
          frame Default {
          }
          frame 0, 5208 {
            n88 = call "Index v0.4.vi"() -> ("error out"=w256:errorcluster)  [unwired: 8 in, 3 out]
          }
        }
        n89 = call-poly "Enqueue Message.vi"("error in (no error)"=w245, "Message"="Check Auto", "Message Queue"=w244) -> ("error out"=w246:errorcluster)  [unwired: 7 in, 1 out]
      }
      frame "Autocycle" {
        n90 = call "Autocycle v0.2.vi"("Message Queue"=w261, "error in"=w264, "Auto Para"=w262) -> ("error out"=w257:errorcluster)  [unwired: 8 in]
        n91 = call-poly "Enqueue Message.vi"("Message Data"=w257, "Message"="Check Auto", "Message Queue"=w258) -> ()  [unwired: 7 in, 2 out]
      }
      frame "Error" {
        n92 = call-poly "Enqueue Message.vi"("error in (no error)"=w267, "Message Data"=w268, "Message"=w269, "Message Queue"=w265) -> ("error out"=w266:errorcluster)  [unwired: 6 in, 1 out]
      }
    }
    n93 = call "Check Loop Error.vi"("Ignore Errors"=i32[] [], "error to process"=w192, "Message Queue"=w184) -> ()  [unwired: 7 in, 2 out]
  }
  n94 = call "Agitator Loop.vi"("error in (no error)"=w9) -> ("error out"=w12:errorcluster)  [unwired: 10 in]
  n95 = call "Bowl Feeder Loop.vi"("error in (no error)"=w9) -> ("error out"=w11:errorcluster)  [unwired: 10 in]
  n96 = call "cRIO-HMI Communication.vi"("error in (no error)"=w9, "Message Queue"=w1) -> ("error out"=w15:errorcluster)  [unwired: 9 in]
  n97 = Merge Errors(w15, w16, w12, w11, w8) -> (w14:errorcluster)
  n98 = xnode ("Close FPGA VI Reference")("FPGA VI Reference In"=w10, "error in"=w14) -> ("error out"=→"error out":errorcluster)
